vi "CRYTime & lot string.vi"(6 "header":enum16{"none", "standard", "custom"}(ring), 8 "Header in":string[][](array[string]), 9 "Lot No.":bool=TRUE, 10 "Time Stamp":bool=TRUE, 11 "Table in":string[][](array[string])) -> (0 "Header out":string[][](array[string]), 1 "Lot string":string, 2 "Time string":string, 3 "Table out":string[][](array[string]))   [LabVIEW 2013]
uses:
  Data/CRYData & result stacks global.vi
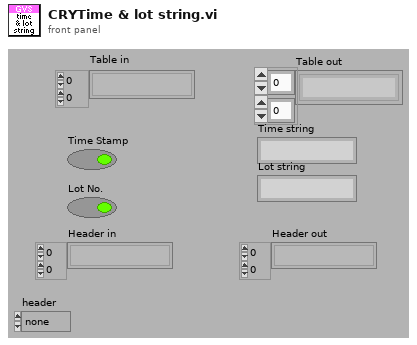
[diagram p1: front panel]
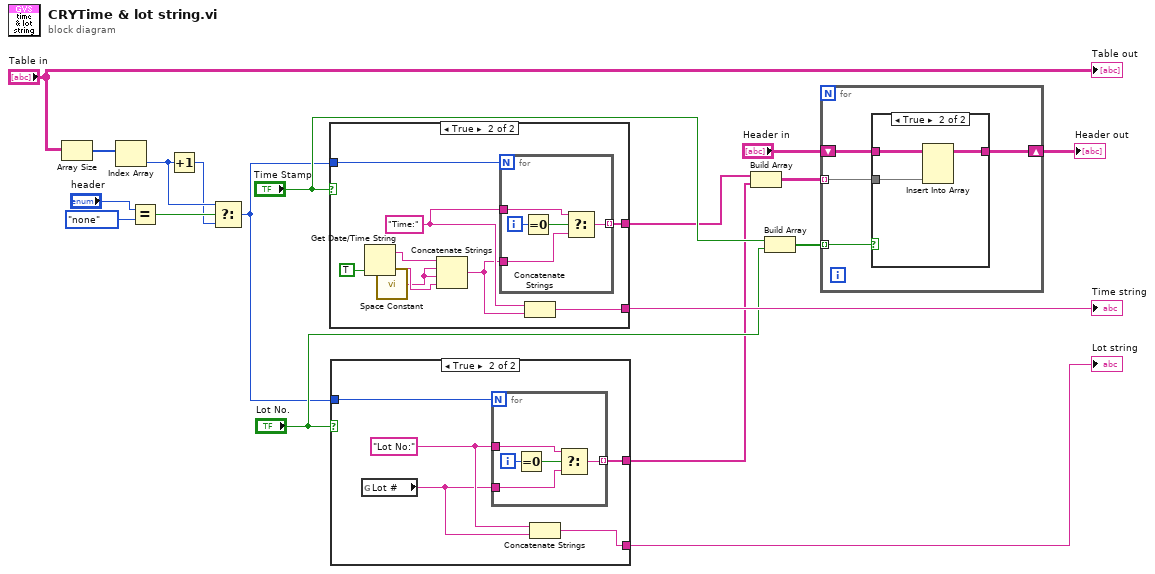
[diagram p0: block diagram]
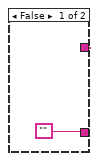
[diagram p3: hidden frame]
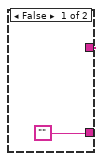
[diagram p4: hidden frame]
diagram:
  n1 = Array Size(array="Table in") -> (size(s)=w18:i32[])
  n2 = Index Array(array=w18) -> (element=w3:i32)  [unwired: 1 in]
  n3 = Equal?(x="header", y=enum16{"none", "standard", "custom"}."none") -> (x = y?=w4:bool)
  n4 = Increment(x=w3) -> (x+1=w2:i32)
  n5 = Select(t=w3, s=w4, f=w2) -> (s? t:f=w1:i32)
  n6 = case shown="True" "Time Stamp" {
    tunnel: w1 -> [_ w28]
    tunnel: [string[] [] w29] -> w9
    tunnel: ["" w21] -> w16
    frame False {
    }
    frame True {
      w23 = "Time:" ("string")
      n7 = Get Date/Time String(want seconds? (F)=TRUE) -> (date string=w24:string, time string=w27:string)  [unwired: 2 in]
      n8 = call <vilib>:"Space Constant.vi"() -> ("String"=w26:string)
      n9 = Concatenate Strings(w24, w26, w26, w27) -> (w22:string)
      n10 = for {
        N: w28 -> [_]
        tunnel: [w33] -> w29 mode=indexing
        tunnel: w23 -> [w31]
        tunnel: w22 -> [w30]
        i -> [w34]
        n11 = Equal To 0?(x=w34) -> (x = 0?=w32:bool)
        n12 = Select(t=w31, s=w32, f=w30) -> (s? t:f=w33:string)
      }
      n13 = Concatenate Strings(w23, w22) -> (w21:string)
    }
  }
  "Time string" <- w16
  n14 = case shown="True" "Lot No." {
    tunnel: w1 -> [_ w40]
    tunnel: [string[] [] w41] -> w8
    tunnel: ["" w37] -> w15
    frame False {
    }
    frame True {
      w39 = "Lot No:" ("string")
      n15 = global read "CRYData & result stacks global.vi" "Lot #"() -> (w38:string)
      n16 = for {
        N: w40 -> [_]
        tunnel: [w45] -> w41 mode=indexing
        tunnel: w39 -> [w43]
        tunnel: w38 -> [w42]
        i -> [w46]
        n17 = Equal To 0?(x=w46) -> (x = 0?=w44:bool)
        n18 = Select(t=w43, s=w44, f=w42) -> (s? t:f=w45:string)
      }
      n19 = Concatenate Strings(w39, w38) -> (w37:string)
    }
  }
  "Lot string" <- w15
  n20 = Build Array(w9, w8) -> (w13:string[][])
  n21 = Build Array("Time Stamp", "Lot No.") -> (w14:bool[])
  n22 = for {
    shift-right: [w47] -> w7
    shift-left: "Header in" -> [w50]
    tunnel: w14 -> [w49] mode=indexing
    tunnel: w13 -> [w48] mode=indexing
    n23 = case shown="True" w49 {
      tunnel: w50 -> [w51 w54]
      tunnel: w48 -> [_ w53]
      tunnel: [w51 w52] -> w47
      frame False {
      }
      frame True {
        n24 = Insert Into Array(array=w54, new element=w53) -> (w52:string[][])  [unwired: 2 in]
      }
    }
  }
  "Header out" <- w7
  "Table out" <- "Table in"
